vi "Read_FromProcessEvent.vi"(8 "error in (no error)":errorcluster, 11 "EVE.lvclass in":refnum<class "EVE.lvclass">) -> (0 "error out":errorcluster, 2 "From Process Event":refnum<user-event>, 3 "EVE.lvclass out":refnum<class "EVE.lvclass">)   [LabVIEW 2013, in "EVE.lvclass"]
uses:
  EVE.lvclass
  030 - EVENTS/05 - FromProcesses/FromProcessEvent.ctl
  030 - EVENTS/05 - FromProcesses/FromProcessesEventType.ctl
  030 - EVENTS/03 - ToMessageHandlerProcess/ToMessageHandlerEvent.ctl
  030 - EVENTS/03 - ToMessageHandlerProcess/enumMessageCriticity.ctl
  EVE.lvclass/EVE.ctl
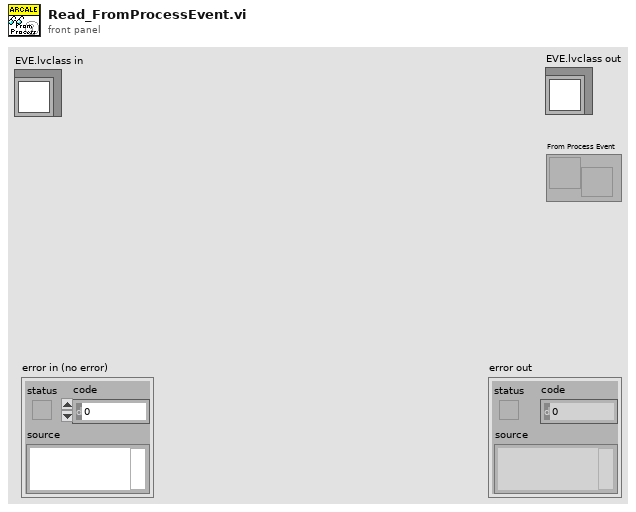
[diagram p1: front panel]
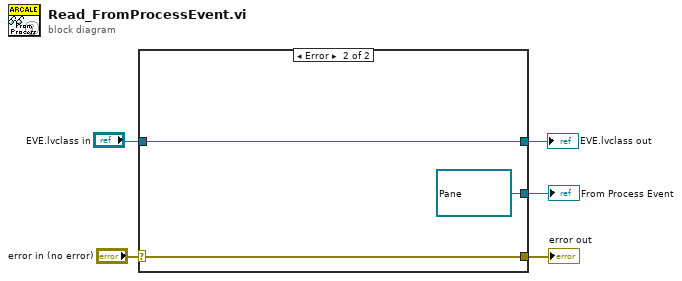
[diagram p0: block diagram]
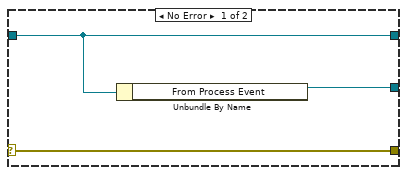
[diagram p2: hidden frame]
diagram:
  n1 = case shown="Error" "error in (no error)" {
    selector: "error in (no error)" -> [w8 w10]
    tunnel: [w8 w10] -> w4
    tunnel: [w6 w11] -> w1
    tunnel: "EVE.lvclass in" -> [w6 w11]
    tunnel: [w7 refnum<user-event> refnum ("From Process Event")] -> w3
    frame No Error {
      n2 = Unbundle By Name(w6) -> ("From Process Event"=w7:refnum<user-event>)
    }
    frame Error {
    }
  }
  "error out" <- w4
  "From Process Event" <- w3
  "EVE.lvclass out" <- w1
